vi "PVCAM_GetDiags.vi"(8 "error in (no error)":errorcluster, 11 "hCam":i16) -> (0 "error out":errorcluster, 2 "return type":i16)   [LabVIEW 2021]
uses:
  Windows/System32/pvcam64.dll
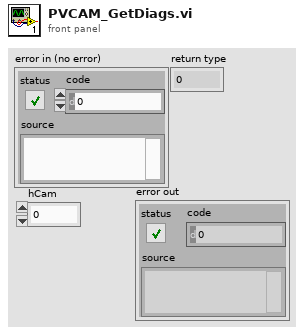
[diagram p1: front panel]
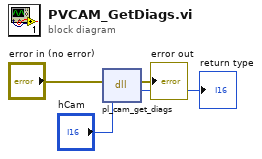
[diagram p0: block diagram]
diagram:
  n1 = dll-call lib="C:/Windows/System32/pvcam64.dll" fn="pl_cam_get_diags"(error in="error in (no error)", "hCam"="hCam") -> (error out=→"error out":errorcluster, "return type"=→"return type":i16)  [unwired: 3 in, 1 out]
